vi "setgain.vi"(8 "error in (no error)":errorcluster, 11 "Imaging in":refnum<class "Imaging.lvclass">) -> (0 "error out":errorcluster, 3 "Imaging out":refnum<class "Imaging.lvclass">)   [LabVIEW 2014, in "Imaging.lvclass"]
uses:
  Imaging.lvclass
  Imaging.lvclass/Imaging.ctl
  <resource>/objmgr/imaqdx.rc
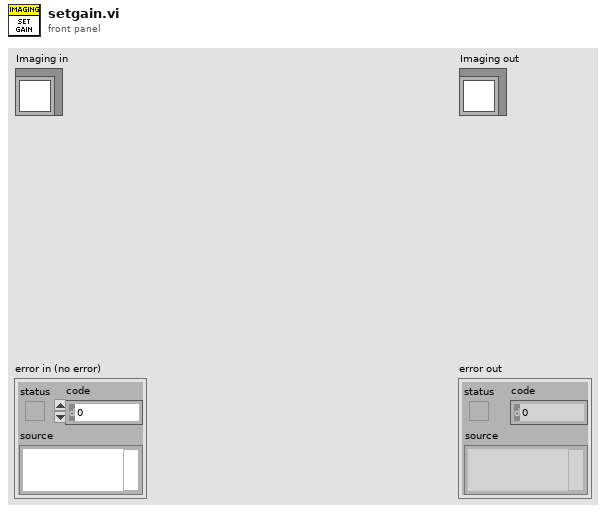
[diagram p1: front panel]
types:
  T1 = typedef "IMAQdx.ctl" = refnum<k21>
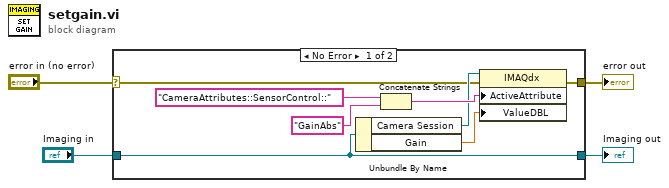
[diagram p0: block diagram]
diagram:
  n1 = case shown="No Error" "error in (no error)" {
    selector: "error in (no error)" -> [w5 w14]
    tunnel: [w8 w13] -> w1
    tunnel: "Imaging in" -> [w8 w13]
    tunnel: [w6 w14] -> w3
    frame No Error {
      n2 = Unbundle By Name(w8) -> ("Camera Session"=w7:T1, "Gain"=w10:dbl)
      n3 = Concatenate Strings("CameraAttributes::SensorControl::" ("string"), "GainAbs" ("string")) -> (w11:string)
      n4 = property class="IMAQdx"(reference=w7, error in=w5, "ActiveAttribute"=w11, "ValueDBL"=w10) -> (error out=w6:errorcluster)  [unwired: 1 out]
    }
    frame Error {
    }
  }
  "error out" <- w3
  "Imaging out" <- w1
